vi "Xeryon serial SendCommand.vi"(3 "error in (no error)":errorcluster, 4 "Feedback?":bool, 5 "Serial Command":T1={"Command"=enum."Exit", "Data to send"=""}) -> (0 "error out":errorcluster, 1 "timed out?":bool, 2 "Feedback":string)   [LabVIEW 2019]
uses:
  Xeryon serial command.ctl
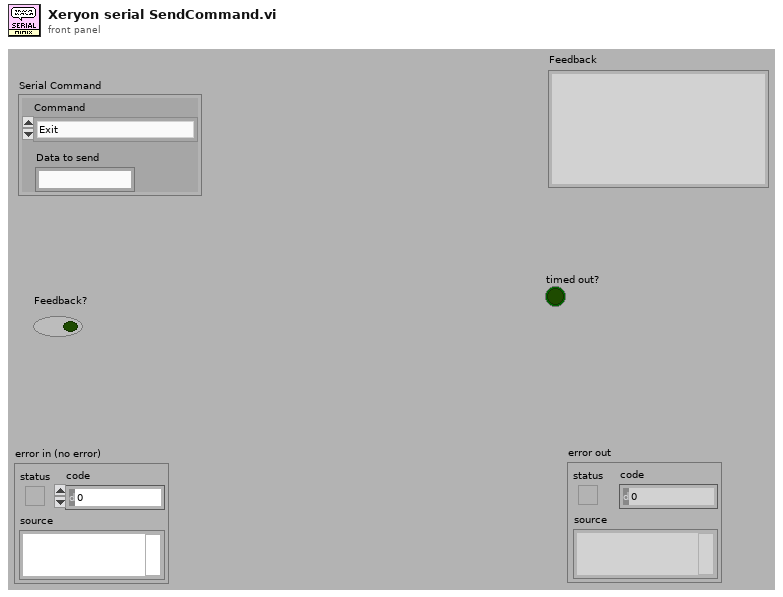
[diagram p1: front panel]
types:
  T1 = typedef "Xeryon serial command.ctl" = cluster{"Command":enum16{"Send serial data", "Exit"}, "Data to send":string}
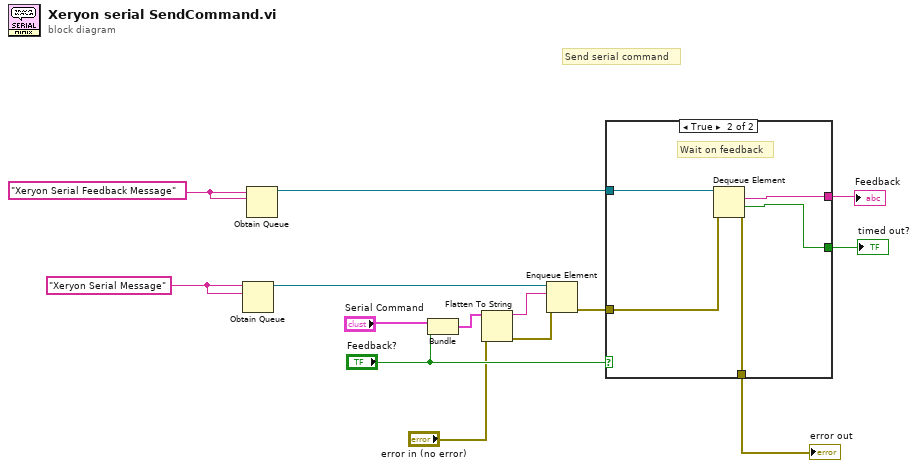
[diagram p0: block diagram]
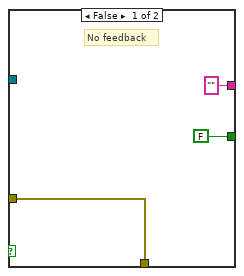
[diagram p2: hidden frame]
diagram:
  w1 = "Xeryon Serial Feedback Message" ("name (unnamed)")
  w2 = "Xeryon Serial Message" ("name (unnamed)")
  # "Send serial command"
  n1 = Obtain Queue(name (unnamed)=w2, element data type=w2) -> (queue out=w8:refnum<queue>)  [unwired: 3 in, 2 out]
  n2 = Obtain Queue(name (unnamed)=w1, element data type=w1) -> (queue out=w12:refnum<queue>)  [unwired: 3 in, 2 out]
  n3 = Bundle("Serial Command"="Serial Command", "Feedback?"="Feedback?") -> (w13:cluster{"Serial Command":T1, "Feedback?":bool})  [unwired: 1 out]
  n4 = Flatten To String(anything=w13, error in (no error)="error in (no error)") -> (data string=w7:string, error out=w4:errorcluster)  [unwired: 3 out]
  n5 = Enqueue Element(queue=w8, element=w7, error in (no error)=w4) -> (error out=w6:errorcluster)  [unwired: 3 out]
  n6 = case shown="True" "Feedback?" {
    tunnel: w12 -> [_ w22]
    tunnel: ["" ("name (unnamed)") w21] -> w11
    tunnel: [FALSE ("timed out?") w20] -> w10
    tunnel: w6 -> [w15 w19]
    tunnel: [w15 w18] -> w3
    frame False {
      # "No feedback"
    }
    frame True {
      # "Wait on feedback"
      n7 = Dequeue Element(queue=w22, error in (no error)=w19) -> (element=w21:string, timed out?=w20:bool, error out=w18:errorcluster)  [unwired: 2 out]
    }
  }
  "timed out?" <- w10
  "Feedback" <- w11
  "error out" <- w3
